vi "Generate Test Data.vi"   [LabVIEW 2020]
types:
  T1 = cluster{"Action":string, "Call Chain":string, "Process":string, "Message":string, "Message Data":variant, "Time":u32}
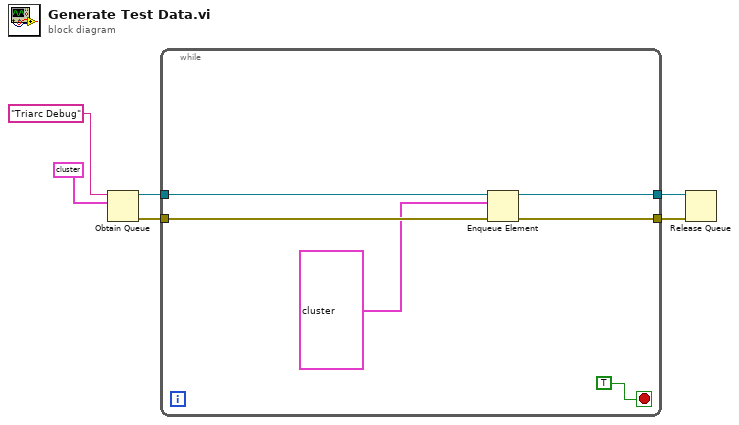
[diagram p0: block diagram]
diagram:
  n1 = Obtain Queue(name (unnamed)="Triarc Debug", element data type=T1 {"Action"="", "Call Chain"="", "Process"="", "Message"="", "Message Data"=variant, "Time"=0} ("output cluster")) -> (queue out=w4:refnum<queue>, error out=w3:errorcluster)  [unwired: 3 in, 1 out]
  n2 = while {
    tunnel: w4 -> [w12]
    tunnel: w3 -> [w9]
    tunnel: [w11] -> w2
    tunnel: [w8] -> w1
    stop <- TRUE ("stop") stop-if-true
    n3 = Enqueue Element(queue=w12, element=T1 {"Action"="Send", "Call Chain"="call chain", "Process"="Process 1", "Message"="Test msg", "Message Data"=variant, "Time"=12}, error in (no error)=w9) -> (queue out=w11:refnum<queue>, error out=w8:errorcluster)  [unwired: 1 in, 1 out]
  }
  n4 = Release Queue(queue=w2, error in (no error)=w1) -> ()  [unwired: 1 in, 3 out]
